vi "CRYNew Graph Cluster.vi"(9 "DataView Number":i32, 10 "Queue Name":string, 11 "Graph Type":string) -> ()   [LabVIEW 2013]
uses:
  Control/CRYGraph Event.ctl
  CRYData View Global.vi
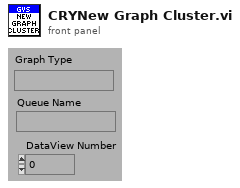
[diagram p1: front panel]
types:
  T1 = typedef "CRYGraph Event.ctl" = cluster{"EvenName":string, "TitleName":string, "GraphName":string, "GraphType":string, "Data":variant, "Queue Name":string, "DataView Number":i32}
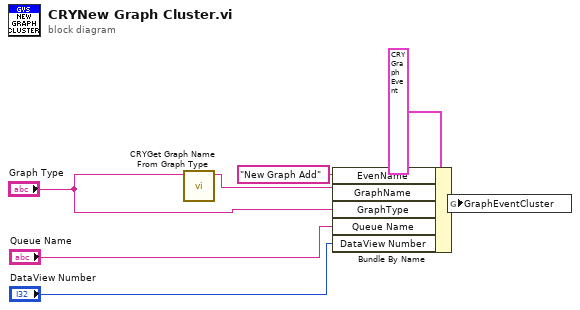
[diagram p0: block diagram]
diagram:
  n1 = call "CRYGet Graph Name From Graph Type.vi"("Graph Type"="Graph Type") -> ("Graph Name"=w2:string)  [unwired: 10 out]
  n2 = Bundle By Name(cluster=T1 {"EvenName"="", "TitleName"="", "GraphName"="", "GraphType"="", "Data"=variant, "Queue Name"="", "DataView Number"=0} ("GraphEventCluster"), "EvenName"="New Graph Add" ("GraphType"), "GraphName"=w2, "GraphType"="Graph Type", "Queue Name"="Queue Name", "DataView Number"="DataView Number") -> (w5:T1)
  n3 = global write "CRYData View Global.vi" "GraphEventCluster"(w5) -> ()
